vi "Drive_Set.vi"   [LabVIEW 2019]
uses:
  Drive_Cluster.ctl
  Drive_States.ctl
  Program Files (x86)/National Instruments/LabVIEW 2019/Targets/NI/RT/vi.lib/Rock Robotics/WPI/DriverStation/WPI_DriverStationRobotMode2.ctl
  Drive_Globals.vi
  Robot Global Data.vi
types:
  T1 = typedef "Drive_Cluster.ctl" = cluster{"Control_State":T2, "Angular_Throttle":dbl, "Linear_Throttle":dbl, "Torque_Changing":bool, "Step":dbl, "Parameter_1":dbl, "Parameter_2":dbl, "Parameter_3":dbl, "Parameter_4":dbl, "Auto_Notifier":refnum<notifier>}
  T2 = typedef "Drive_States.ctl" = enum16{"Percent_Voltage_Control", "Speed_Control", "Command_HeadingDistance", "Command_TurnToHeading"}
  T3 = typedef "WPI_DriverStationRobotMode2.ctl" = enum16{"Autonomous Disabled", "Autonomous Enabled", "Teleop Disabled", "Teleop Enabled", "Disconnected", "Finish", "Test Disabled", "Test Enabled", "Emergency Stopped"}
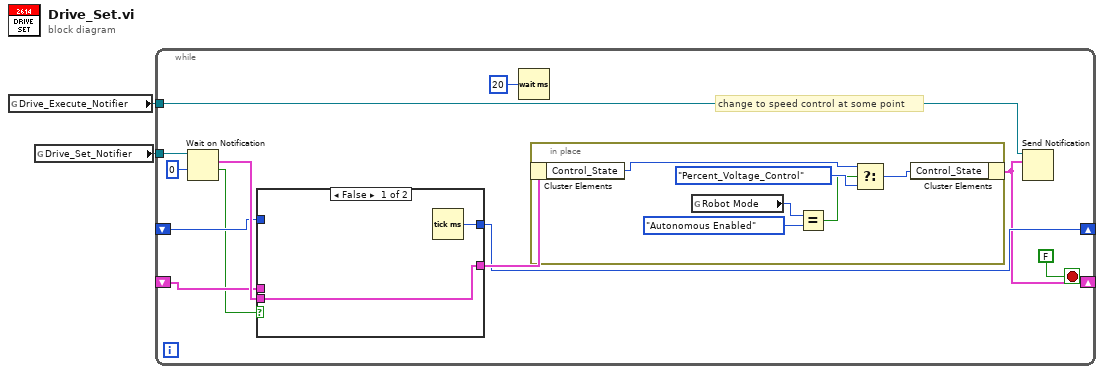
[diagram p0: block diagram]
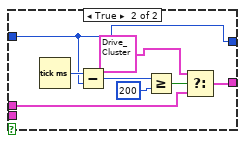
[diagram p2: hidden frame]
diagram:
  n1 = global read "Drive_Globals.vi" "Drive_Execute_Notifier"() -> (w1:refnum<notifier>)
  n2 = global read "Drive_Globals.vi" "Drive_Set_Notifier"() -> (w2:refnum<notifier>)
  n3 = while {
    tunnel: w2 -> [w13]
    tunnel: w1 -> [w12]
    shift-right: [w8] -> _
    shift-left: _ -> [w7]
    shift-right: [w6] -> _
    shift-left: _ -> [w5]
    stop <- FALSE stop-if-true
    # "change to speed control at some point"
    n4 = Wait on Notification(notifier=w13, timeout in ms (-1)=0) -> (notification=w9:T1, timed out?=w4:bool)  [unwired: 2 in, 2 out]
    n5 = case shown="False" w4 {
      tunnel: w9 -> [w16 _]
      tunnel: [w16 w19] -> w10
      tunnel: [w15 w23] -> w8
      tunnel: w7 -> [_ w23]
      tunnel: w5 -> [_ w17]
      frame False {
        n6 = Tick Count (ms)() -> (millisecond timer value=w15:u32)
      }
      frame True {
        n7 = Tick Count (ms)() -> (millisecond timer value=w24:u32)
        n8 = Subtract(x=w24, y=w23) -> (x-y=w22:u32)
        n9 = Greater Or Equal?(x=w22, y=u32 200) -> (x >= y?=w20:bool)
        n10 = Select(t=T1 {"Control_State"=enum."Percent_Voltage_Control", "Angular_Throttle"=0.0, "Linear_Throttle"=0.0, "Torque_Changing"=FALSE, "Step"=0.0, "Parameter_1"=0.0, "Parameter_2"=0.0, "Parameter_3"=0.0, "Parameter_4"=0.0, "Auto_Notifier"=refnum} ("Drive_Cluster"), s=w20, f=w17) -> (s? t:f=w19:T1)
      }
    }
    n11 = Wait (ms)(milliseconds to wait=u32 20) -> ()  [unwired: 1 out]
    n12 = in-place {
      n13 = in-place-cluster #1(w10) -> ("Control_State"=w26:T2)
      n14 = global read "Robot Global Data.vi" "Robot Mode"() -> (w28:T3)
      n15 = Equal?(x=w28, y=WPI_DriverStationRobotMode2."Autonomous Enabled") -> (x = y?=w25:bool)
      n16 = Select(t=w26, s=w25, f=Drive_States."Percent_Voltage_Control" ("Control_State")) -> (s? t:f=w30:T2)
      n17 = in-place-cluster #1("Control_State"=w30) -> (w6:T1)
    }
    n18 = Send Notification(notification=w6, notifier=w12) -> ()  [unwired: 1 in, 2 out]
  }
